vi "HFRR ADV v06.vi"() -> ()   [LabVIEW 2025] (continued)
            n239 = Concatenate Strings("[CH3]" ("string"), w309, " - 20x Gain" ("string"), "\r") -> (w303:string)
            n240 = Concatenate Strings("[CH4]" ("string"), w297, " - 100x Gain" ("string"), "\r") -> (w296:string)
            n241 = String To Path(string="C:\\LAB-IQ\\Image Calibrate v01.dcf") -> (path=w326:path)
            n242 = Concatenate Strings(w313, w312, w303, w296) -> (w311:string)
            n243 = call <vilib>:"Write Characters To File.vi"("append to file? (new file:F)"=FALSE, "character string"=w311, "file path (dialog if empty)"=w326) -> ()  [unwired: 2 in, 1 out]
          }
          frame #2 {
            n244 = String To Path(string="C:\\LAB-IQ\\Image Calibrate v01.dcf") -> (path=w329:path)
            n245 = Open/Create/Replace File ("Open File")(file path (use dialog)=w329) -> (refnum out=w330:refnum<file>)  [unwired: 5 in, 2 out]
            n246 = for {
              N: 4 -> [_]
              tunnel: w330 -> [w336]
              i -> [w332]
              n247 = Read from Text File ("Read File")(file (use dialog)=w336) -> (text=w337:string)  [unwired: 3 in, 3 out]
              n248 = String Subset(string=w337, offset (0)=6, length (rest)=10 ("length (rest)")) -> (substring=w333:string)
              n249 = Fract/Exp String To Number(string=w333) -> (number=w331:dbl)  [unwired: 3 in, 1 out]
              n250 = case shown="3" w332 {
                tunnel: w331 -> [w338 w339 _ w340 _]
                frame 0 {
                  n251 = local write "5x Gain"(w338) -> ()
                }
                frame 1 {
                  n252 = local write "10x Gain"(w339) -> ()
                }
                frame 2 {
                }
                frame 3 {
                  n253 = local write "100x gain"(w340) -> ()
                }
                frame 4, Default {
                }
              }
            }
          }
          frame #3 {
            n254 = call "IMAGE ANALYSIS.vi"("Enum"=POST_ANALYSIS_ENUM."SHOW UI") -> ()  [unwired: 9 in, 2 out]
          }
          frame #4 {
            n255 = Not(x=w343) -> (.not. x?=w342:bool)
            n256 = local write "Save Change"(w342) -> ()
          }
        }
      }
    }
    n257 = local read "Cap Live Image"() -> (w269:bool)
    n258 = local read "SCAR MEASURMENT"() -> (w272:enum32{"Auto Scar", "Manual Scar"})
    n259 = Wait (ms)(milliseconds to wait=u32 250) -> ()  [unwired: 1 out]
    n260 = Equal?(x=w272, y=enum32{"Auto Scar", "Manual Scar"}."Manual Scar" ("SCAR MEASURMENT")) -> (x = y?=w270:bool)
    n261 = And(x=w270, y=w269) -> (x .and. y?=w268:bool)
    n262 = case shown="True" w268 {
      selector: w268 -> [_ w536]
      frame False {
      }
      frame True {
        n263 = stacked-sequence {
          tunnel: [_ _ _ w551 _] -> _
          tunnel: w536 -> [_ _ _ _ w557]
          frame #0 {
            w537 = 0.0
            n264 = local write "Major Axis"(w537) -> ()
            n265 = local write "Minor Axis"(w537) -> ()
            n266 = local write "Average"(w537) -> ()
          }
          frame #1 {
            n267 = call "CAMERA LIVE FEED FGV.vi"("Enum - Menu"=CAMERA_LIVE_FEED_ENUM."CAMERA MINIMIZE") -> ()  [unwired: 9 in, 2 out]
          }
          frame #2 {
            n268 = local read "FILE 3"() -> (w545:string)
            n269 = call <vilib>:"Trim Whitespace.vi"("string"="C:\\LAB-IQ\\images\\") -> ("trimmed string"=w547:string)  [unwired: 1 in]
            n270 = String To Path(string=w547) -> (path=w546:path)
            n271 = Concatenate Strings(w545, ".png" ("string")) -> (w544:string)
            n272 = Build Path(base path=w546, name or relative path=w544) -> (appended path=w542:path)
            n273 = Path To String(path=w542) -> (string=w541:string)
            n274 = call "CAMERA LIVE FEED FGV.vi"("Enum - Menu"=CAMERA_LIVE_FEED_ENUM."CAMERA SAVE", "Image Path"=w541) -> ("error out"=w539:errorcluster)  [unwired: 8 in, 1 out]
            n275 = case shown="No Error" w539 {
              frame No Error {
                n276 = One Button Dialog(message="Image saved successfully") -> ()  [unwired: 1 in, 1 out]
              }
              frame Error {
              }
            }
          }
          frame #3 {
            n277 = call "LIST FILE NAMES.vi"() -> ("error out"=w553:errorcluster, "filenames"=w550:string[])  [unwired: 10 in]
            n278 = call "IMAGE ANALYSIS.vi"("Enum"=POST_ANALYSIS_ENUM."SHOW UI", "error in"=w553) -> ("error out"=w551:errorcluster)  [unwired: 8 in, 1 out]
            n279 = property on="Test File List :" class="CmbBox"("Strings[]"=w550) -> ()  [unwired: 2 in, 2 out]
          }
          frame #4 {
            n280 = Not(x=w557) -> (.not. x?=w556:bool)
            n281 = local write "Zoom Factore"(0.0 ("Zoom Factore")) -> ()
            n282 = local write "Cap Live Image"(w556) -> ()
            n283 = local write "Main Tab"(T2."Adv Scar Report" ("Main Tab")) -> ()
            n284 = local write "Main Dashboard Buttons"(T1."Report" ("Main Dashboard Buttons")) -> ()
            n285 = property on="Cap Live Image" class="Bool (strict)"("BoolText.Text"="Capture Image" ("Boolean Text.Text")) -> ()  [unwired: 2 in, 2 out]
          }
        }
      }
    }
    n286 = local read "change Gain"() -> (w252:bool)
    n287 = local read "Back Square"() -> (w251:bool)
    n288 = case shown="True" w252 {
      selector: w252 -> [_ w280]
      frame False {
      }
      frame True {
        n289 = stacked-sequence {
          tunnel: w280 -> [_ w288]
          frame #0 {
            n290 = local read "Actual (µm)"() -> (w284:dbl)
            n291 = local read "Pixel Value"() -> (w283:dbl)
            n292 = local read "Magnification :"() -> (w282:string)
            n293 = Divide(x=w284, y=w283) -> (x/y=w281:dbl)
            n294 = case shown="\"10x\"" w282 {
              tunnel: w281 -> [w285 w286]
              frame "10x" {
                n295 = local write "10x Gain"(w285) -> ()
              }
              frame "5x", Default {
                n296 = local write "5x Gain"(w286) -> ()
              }
            }
          }
          frame #1 {
            n297 = Not(x=w288) -> (.not. x?=w287:bool)
            n298 = local write "change Gain"(w287) -> ()
          }
        }
      }
    }
    n299 = case shown="True" w251 {
      selector: w251 -> [_ w278]
      frame False {
      }
      frame True {
        n300 = Not(x=w278) -> (.not. x?=w277:bool)
        n301 = local write "Back Square"(w277) -> ()
        n302 = local write "Calibration Tab"(enum32{"Measrument", "Calibrate"}."Measrument" ("Calibration Tab")) -> ()
      }
    }
    n303 = local read "Rectangle Tool"() -> (w263:bool)
    n304 = local read "Clear ROI Tool"() -> (w262:bool)
    n305 = local read "Open Image"() -> (w267:bool)
    n306 = local read "line tool"() -> (w264:bool)
    n307 = local read "OUT"() -> (w265:bool)
    n308 = local read "In"() -> (w266:bool)
    n309 = case shown="True" w267 {
      selector: w267 -> [_ w524]
      tunnel: [w520 w526] -> _
      tunnel: w257 -> [w520 w525]
      frame False {
      }
      frame True {
        n310 = Not(x=w524) -> (.not. x?=w523:bool)
        n311 = local write "Open Image"(w523) -> ()
        n312 = call "IMAGE ANALYSIS.vi"("Enum"=POST_ANALYSIS_ENUM."HIDE UI", "error in"=w525) -> ("error out"=w533:errorcluster)  [unwired: 8 in, 1 out]
        n313 = call "File Dialog"("start path"=path "C:/LAB-IQ/images", "error in"=w533) -> ("selected path"=w522:path, "error out"=w531:errorcluster)  [unwired: 10 in, 2 out]
        "Image path" <- w522
        n314 = call <vilib>:"Clear Errors.vi"("error in (no error)"=w531) -> ("error out"=w530:errorcluster)  [unwired: 5 in, 1 out]
        n315 = call "IMAGE ANALYSIS.vi"("Enum"=POST_ANALYSIS_ENUM."OPEN FILE", "error in"=w530, "File Path"=w522) -> ("error out"=w529:errorcluster)  [unwired: 7 in, 1 out]
        n316 = call <vilib>:"Clear Errors.vi"("error in (no error)"=w529) -> ("error out"=w528:errorcluster)  [unwired: 5 in, 1 out]
        n317 = call "IMAGE ANALYSIS.vi"("Enum"=POST_ANALYSIS_ENUM."SHOW UI", "error in"=w528) -> ("error out"=w526:errorcluster)  [unwired: 8 in, 1 out]
        n318 = local write "Zoom Factore"(100.0 ("Zoom Factore")) -> ()
      }
    }
    n319 = case shown="True" w265 {
      selector: w265 -> [_ w505]
      tunnel: w257 -> [w502 w510]
      tunnel: [w502 w504] -> _
      frame False {
      }
      frame True {
        n320 = Not(x=w505) -> (.not. x?=w503:bool)
        n321 = local read "Zoom Factore"() -> (w508:dbl)
        n322 = local write "OUT"(w503) -> ()
        n323 = call "IMAGE ANALYSIS.vi"("Enum"=POST_ANALYSIS_ENUM."ZOOM OUT", "error in"=w510) -> ("error out"=w504:errorcluster)  [unwired: 8 in, 1 out]
        n324 = Divide(x=w508, y=1.2) -> (x/y=w506:dbl)
        n325 = local write "Zoom Factore"(w506) -> ()
      }
    }
    n326 = case shown="True" w266 {
      selector: w266 -> [_ w514]
      tunnel: w257 -> [w511 w519]
      tunnel: [w511 w512] -> _
      frame False {
      }
      frame True {
        n327 = Not(x=w514) -> (.not. x?=w513:bool)
        n328 = local read "Zoom Factore"() -> (w517:dbl)
        n329 = local write "In"(w513) -> ()
        n330 = call "IMAGE ANALYSIS.vi"("Enum"=POST_ANALYSIS_ENUM."ZOOM IN", "error in"=w519) -> ("error out"=w512:errorcluster)  [unwired: 8 in, 1 out]
        n331 = Multiply(x=w517, y=1.2) -> (x*y=w515:dbl)
        n332 = local write "Zoom Factore"(w515) -> ()
      }
    }
    n333 = case shown="True" w262 {
      selector: w262 -> [_ w486]
      tunnel: w257 -> [w484 w488]
      tunnel: [w484 w487] -> _
      frame False {
      }
      frame True {
        n334 = Not(x=w486) -> (.not. x?=w485:bool)
        n335 = local write "Clear ROI Tool"(w485) -> ()
        n336 = call "IMAGE ANALYSIS.vi"("Enum"=POST_ANALYSIS_ENUM."CLEAR ROI", "error in"=w488) -> ("error out"=w487:errorcluster)  [unwired: 8 in, 1 out]
      }
    }
    n337 = case shown="True" w264 {
      selector: w264 -> [_ w498]
      tunnel: w257 -> [w496 w501]
      tunnel: [w496 w499] -> _
      frame False {
      }
      frame True {
        n338 = Not(x=w498) -> (.not. x?=w497:bool)
        n339 = local write "line tool"(w497) -> ()
        n340 = call "IMAGE ANALYSIS.vi"("Enum"=POST_ANALYSIS_ENUM."DRAW LINE", "error in"=w501) -> ("error out"=w499:errorcluster)  [unwired: 8 in, 1 out]
      }
    }
    n341 = case shown="True" w263 {
      selector: w263 -> [_ w492]
      tunnel: w257 -> [w490 w494]
      tunnel: [w490 w493] -> _
      frame False {
      }
      frame True {
        n342 = Not(x=w492) -> (.not. x?=w491:bool)
        n343 = local write "Rectangle Tool"(w491) -> ()
        n344 = call "IMAGE ANALYSIS.vi"("Enum"=POST_ANALYSIS_ENUM."DRAW REC", "error in"=w494) -> ("error out"=w493:errorcluster)  [unwired: 8 in, 1 out]
      }
    }
    n345 = local read "SCAR MEASURMENT"() -> (w250:enum32{"Auto Scar", "Manual Scar"})
    n346 = local read "Fit to Screen Tool"() -> (w259:bool)
    n347 = local read "Resize Tool"() -> (w258:bool)
    n348 = case shown="\"Manual Scar\"" w250 {
      frame "Auto Scar", Default {
        n349 = property on="Cap Live Image" class="Bool (strict)"("BoolText.Text"="Report" ("Boolean Text.Text")) -> ()  [unwired: 2 in, 2 out]
      }
      frame "Manual Scar" {
        n350 = property on="Cap Live Image" class="Bool (strict)"("BoolText.Text"="Save Image" ("Boolean Text.Text")) -> ()  [unwired: 2 in, 2 out]
      }
    }
    n351 = local read "ROI Color Tool"() -> (w260:bool)
    n352 = local read "Pan Tool"() -> (w261:bool)
    n353 = case shown="True" w261 {
      selector: w261 -> [_ w480]
      tunnel: w257 -> [w478 w482]
      tunnel: [w478 w481] -> _
      frame False {
      }
      frame True {
        n354 = Not(x=w480) -> (.not. x?=w479:bool)
        n355 = call "IMAGE ANALYSIS.vi"("Enum"=POST_ANALYSIS_ENUM."PAN", "error in"=w482) -> ("error out"=w481:errorcluster)  [unwired: 8 in, 1 out]
        n356 = local write "Pan Tool"(w479) -> ()
      }
    }
    n357 = case shown="True" w258 {
      selector: w258 -> [_ w464]
      tunnel: w257 -> [w459 w461]
      tunnel: [w459 w460] -> _
      frame False {
      }
      frame True {
        n358 = Not(x=w464) -> (.not. x?=w463:bool)
        n359 = local write "Resize Tool"(w463) -> ()
        n360 = call "IMAGE ANALYSIS.vi"("Enum"=POST_ANALYSIS_ENUM."RESIZE MODE", "error in"=w461) -> ("error out"=w460:errorcluster)  [unwired: 8 in, 1 out]
      }
    }
    n361 = case shown="True" w259 {
      selector: w259 -> [_ w469]
      tunnel: [w465 w470] -> _
      tunnel: w257 -> [w465 w468]
      frame False {
      }
      frame True {
        n362 = Not(x=w469) -> (.not. x?=w467:bool)
        n363 = local write "Zoom Factore"(100.0 ("Zoom Factore")) -> ()
        n364 = local write "Fit to Screen Tool"(w467) -> ()
        n365 = call "IMAGE ANALYSIS.vi"("Enum"=POST_ANALYSIS_ENUM."FIT", "error in"=w468) -> ("error out"=w470:errorcluster)  [unwired: 8 in, 1 out]
      }
    }
    n366 = case shown="True" w260 {
      selector: w260 -> [_ w475]
      tunnel: [w472 w476] -> _
      tunnel: w257 -> [w472 w473]
      frame False {
      }
      frame True {
        n367 = Not(x=w475) -> (.not. x?=w474:bool)
        n368 = local write "ROI Color Tool"(w474) -> ()
        n369 = call "IMAGE ANALYSIS.vi"("Enum"=POST_ANALYSIS_ENUM."SET ROI COLOR", "error in"=w473) -> ("error out"=w476:errorcluster)  [unwired: 8 in, 1 out]
      }
    }
    n370 = local read "Quit"() -> (w274:bool)
  }
  n371 = property on="Auto Scar Check  2" class="Clust (strict)"("Visible"=FALSE) -> (error out=w1:errorcluster)  [unwired: 2 in, 1 out]
  n372 = while {
    stop <- w560 stop-if-true
    n373 = local read "Image Path"() -> (w563:path)
    n374 = local read "Print 3"() -> (w566:bool)
    n375 = Equal?(x=w563, y=path "") -> (x = y?=w562:bool)
    n376 = Not(x=w562) -> (.not. x?=w561:bool)
    n377 = property on="Print 3" class="Bool (strict)"("Visible"=w561) -> ()  [unwired: 2 in, 2 out]
    n378 = case shown="True" w566 {
      frame False {
        n379 = local write "Rd"(TRUE ("Boolean 7")) -> ()
      }
      frame True {
        n380 = flat-sequence {
          tunnel: [w606] -> w574
          tunnel: [w593] -> w572
          tunnel: [w603] -> w568
          tunnel: w574 -> [w615]
          tunnel: [w615] -> w573
          tunnel: w572 -> [w614]
          tunnel: [w614] -> w571
          tunnel: [w612] -> w570
          tunnel: [w611] -> w569
          tunnel: w568 -> [w611]
          tunnel: w573 -> [w617]
          tunnel: w571 -> [w618]
          tunnel: w570 -> [_]
          tunnel: w569 -> [w616]
          frame #0 {
            n381 = case shown="True" "Rd" {
              frame False {
              }
              frame True {
                n382 = while {
                  tunnel: "abcdefABCDEF" ("string 2") -> [w585]
                  shift-right: [w583] -> w577
                  shift-left: "" -> [w582]
                  i -> [w592]
                  stop <- w591 stop-if-true
                  n383 = Random Number (0-1)() -> (number: 0 to 1=w586:dbl)
                  n384 = Multiply(x=w586, y=62.0) -> (x*y=w588:dbl)
                  n385 = Decrement(x="Length 2") -> (x-1=w581:i16)
                  n386 = To Word Integer(number=w588) -> (16bit integer=w589:i16)
                  n387 = String Subset(string=w585, offset (0)=w589, length (rest)=1 ("length (rest)")) -> (substring=w584:string)
                  n388 = Greater Or Equal?(x=w592, y=w581) -> (x >= y?=w591:bool)
                  n389 = Concatenate Strings(w584, w582) -> (w583:string)
                }
                "String 10" <- w577
                n390 = local write "Rd"(FALSE ("Boolean 7")) -> ()
              }
            }
          }
          frame #1 {
            w604 = "_resized.jpg" ("command line")
            (unwired) ".jpg -resize 320x240 " ("string")
            (unwired) "Choose an Image File" ("prompt")
            # "-resize 1798x425"
            n391 = local read "Image Path"() -> (w598:path)
            n392 = Strip Path(path=w598) -> (stripped path=w593:path, name=w594:string)
            n393 = Match Pattern(string=w594, regular expression=".jpg") -> (before substring=→"before substring 2":string, after substring=→"after substring":string)  [unwired: 1 in, 2 out]
            n394 = Match Pattern(string=w594, regular expression="\\") -> (before substring=w600:string)  [unwired: 1 in, 3 out]
            n395 = Match Pattern(string=w600, regular expression=".jpg") -> (before substring=w599:string)  [unwired: 1 in, 3 out]
            n396 = Concatenate Strings("cmd /c convert " ("string"), w599, ".jpg -resize 320x240  " ("command line"), w599, w604) -> (w607:string)
            n397 = call <vilib>:"System Exec.vi"("run minimized? (F)"=TRUE, "wait until completion? (T)"=TRUE, "working directory"=w593, "command line"=w607) -> ("error out"=w606:errorcluster)  [unwired: 4 in, 3 out]
            "error out 2" <- w606
            n398 = Concatenate Strings(w599, w604) -> (w603:string)
          }
          frame #2 {
            n399 = Wait (ms)(milliseconds to wait=u32 2000 ("millisecond timer value")) -> (millisecond timer value=w612:u32)
          }
          frame #3 {
            n400 = case shown="No Error" w617 {
              tunnel: w618 -> [w621 _]
              tunnel: w616 -> [w619 _]
              frame No Error {
                (unwired) ".jpg" ("string")
                n401 = Path To String(path=w621) -> (string=w625:string)
                n402 = Concatenate Strings(w625, "\\" ("string"), w619) -> (w624:string)
                n403 = String To Path(string=w624) -> (path=w623:path)
                n404 = call <vilib>:"Read JPEG File.vi"("path to JPEG file"=w623) -> ("image data"=w627:T11)  [unwired: 8 in, 2 out]
                "image data" <- w627
                n405 = local write "Print 3"(FALSE ("Print 2")) -> ()
                n406 = call <vilib>:"Draw Flattened Pixmap.vi"("image data"=w627) -> ("new picture"=→"new picture":picture)  [unwired: 8 in]
              }
              frame Error {
              }
            }
          }
        }
      }
    }
    n407 = Wait (ms)(milliseconds to wait=u32 20 ("millisecond timer value")) -> ()  [unwired: 1 out]
    n408 = local read "Quit"() -> (w560:bool)
  }
  n409 = while {
    tunnel: w21 -> [_]
    tunnel: w1 -> [_]
    stop <- w657 stop-if-true
    # "New Adv Logics"
    n410 = local read "Main Tab"() -> (w655:T2)
    n411 = local read "Sign In"() -> (w654:bool)
    n412 = local read "Main Tab"() -> (w636:T2)
    n413 = case shown="\"Adv Scar Report\"" w636 {
      frame "HOME", Default {
        n414 = local read "LIVE FEED MIN TEMP"() -> (w726:bool)
        n415 = local write "LIVE FEED MAX TEMP"(TRUE ("LIVE FEED MAX TEMP")) -> ()
        n416 = local read "CAMERA ROI MIN TEMP"() -> (w724:bool)
        n417 = case shown="True" w726 {
          selector: w726 -> [_ w733]
          frame False {
          }
          frame True {
            n418 = Not(x=w733) -> (.not. x?=w732:bool)
            n419 = local write "LIVE FEED MIN TEMP"(w732) -> ()
            n420 = call "CAMERA LIVE FEED FGV.vi"("Enum - Menu"=CAMERA_LIVE_FEED_ENUM."CAMERA MINIMIZE") -> ()  [unwired: 9 in, 2 out]
          }
        }
        n421 = case shown="True" w724 {
          selector: w724 -> [_ w730]
          frame False {
          }
          frame True {
            n422 = Not(x=w730) -> (.not. x?=w729:bool)
            n423 = local write "CAMERA ROI MIN TEMP"(w729) -> ()
            n424 = call "IMAGE ANALYSIS.vi"("Enum"=POST_ANALYSIS_ENUM."MINIMIZE UI") -> ()  [unwired: 9 in, 2 out]
          }
        }
        n425 = local write "CAMERA ROI MAX TEMP"(TRUE ("CAMERA ROI MAX TEMP")) -> ()
      }
      frame "Test Setup" {
        n426 = local read "LIVE FEED MIN TEMP"() -> (w736:bool)
        n427 = local read "CAMERA ROI MIN TEMP"() -> (w734:bool)
        n428 = local write "LIVE FEED MAX TEMP"(TRUE ("LIVE FEED MAX TEMP")) -> ()
        n429 = case shown="True" w736 {
          selector: w736 -> [_ w743]
          frame False {
          }
          frame True {
            n430 = Not(x=w743) -> (.not. x?=w742:bool)
            n431 = local write "LIVE FEED MIN TEMP"(w742) -> ()
            n432 = call "CAMERA LIVE FEED FGV.vi"("Enum - Menu"=CAMERA_LIVE_FEED_ENUM."CAMERA MINIMIZE") -> ()  [unwired: 9 in, 2 out]
          }
        }
        n433 = case shown="True" w734 {
          selector: w734 -> [_ w740]
          frame False {
          }
          frame True {
            n434 = Not(x=w740) -> (.not. x?=w739:bool)
            n435 = local write "CAMERA ROI MIN TEMP"(w739) -> ()
            n436 = call "IMAGE ANALYSIS.vi"("Enum"=POST_ANALYSIS_ENUM."MINIMIZE UI") -> ()  [unwired: 9 in, 2 out]
          }
        }
        n437 = local write "CAMERA ROI MAX TEMP"(TRUE ("CAMERA ROI MAX TEMP")) -> ()
      }
      frame "Acquire" {
        n438 = local read "LIVE FEED MIN TEMP"() -> (w746:bool)
        n439 = local write "LIVE FEED MAX TEMP"(TRUE ("LIVE FEED MAX TEMP")) -> ()
        n440 = local read "CAMERA ROI MIN TEMP"() -> (w744:bool)
        n441 = case shown="True" w746 {
          selector: w746 -> [_ w753]
          frame False {
          }
          frame True {
            n442 = Not(x=w753) -> (.not. x?=w752:bool)
            n443 = local write "LIVE FEED MIN TEMP"(w752) -> ()
            n444 = call "CAMERA LIVE FEED FGV.vi"("Enum - Menu"=CAMERA_LIVE_FEED_ENUM."CAMERA MINIMIZE") -> ()  [unwired: 9 in, 2 out]
          }
        }
        n445 = case shown="True" w744 {
          selector: w744 -> [_ w750]
          frame False {
          }
          frame True {
            n446 = Not(x=w750) -> (.not. x?=w749:bool)
            n447 = local write "CAMERA ROI MIN TEMP"(w749) -> ()
            n448 = call "IMAGE ANALYSIS.vi"("Enum"=POST_ANALYSIS_ENUM."MINIMIZE UI") -> ()  [unwired: 9 in, 2 out]
          }
        }
        n449 = local write "CAMERA ROI MAX TEMP"(TRUE ("CAMERA ROI MAX TEMP")) -> ()
      }
      frame "Adv Scar" {
        n450 = local read "CAMERA ROI MIN TEMP"() -> (w754:bool)
        n451 = case shown="True" "LIVE FEED MAX TEMP" {
          selector: "LIVE FEED MAX TEMP" -> [_ w766]
          frame False {
          }
          frame True {
            n452 = Not(x=w766) -> (.not. x?=w765:bool)
            n453 = local write "LIVE FEED MAX TEMP"(w765) -> ()
            n454 = call "CAMERA LIVE FEED FGV.vi"("Enum - Menu"=CAMERA_LIVE_FEED_ENUM."CAMERA RESTORE") -> ("error out"=w761:errorcluster)  [unwired: 9 in, 1 out]
            n455 = call "LIST FILE NAMES.vi"("error in (no error)"=w761) -> ("error out"=w762:errorcluster, "filenames"=w763:string[])  [unwired: 9 in]
            n456 = property on="FILE 3" class="CmbBox"(error in=w762, "Strings[]"=w763) -> ()  [unwired: 1 in, 2 out]
          }
        }
        n457 = case shown="True" w754 {
          selector: w754 -> [_ w760]
          frame False {
          }
          frame True {
            n458 = Not(x=w760) -> (.not. x?=w759:bool)
            n459 = local write "CAMERA ROI MIN TEMP"(w759) -> ()
            n460 = call "IMAGE ANALYSIS.vi"("Enum"=POST_ANALYSIS_ENUM."MINIMIZE UI") -> ()  [unwired: 9 in, 2 out]
          }
        }
        n461 = local write "CAMERA ROI MAX TEMP"(TRUE ("CAMERA ROI MAX TEMP")) -> ()
        "LIVE FEED MIN TEMP" <- TRUE ("LIVE FEED MIN TEMP")
      }
      frame "Adv Scar Report" {
        n462 = local read "CAMERA ROI MAX TEMP"() -> (w767:bool)
        n463 = local read "LIVE FEED MIN TEMP"() -> (w769:bool)
        n464 = local write "LIVE FEED MAX TEMP"(TRUE ("LIVE FEED MAX TEMP")) -> ()
        n465 = case shown="True" w769 {
          selector: w769 -> [_ w778]
          frame False {
          }
          frame True {
            n466 = Not(x=w778) -> (.not. x?=w777:bool)
            n467 = local write "LIVE FEED MIN TEMP"(w777) -> ()
            n468 = call "CAMERA LIVE FEED FGV.vi"("Enum - Menu"=CAMERA_LIVE_FEED_ENUM."CAMERA MINIMIZE") -> ()  [unwired: 9 in, 2 out]
          }
        }
        n469 = case shown="True" w767 {
          selector: w767 -> [_ w775]
          frame False {
          }
          frame True {
            n470 = Not(x=w775) -> (.not. x?=w773:bool)
            n471 = local write "CAMERA ROI MAX TEMP"(w773) -> ()
            n472 = call "IMAGE ANALYSIS.vi"("Enum"=POST_ANALYSIS_ENUM."SHOW UI") -> ("error out"=w772:errorcluster)  [unwired: 9 in, 1 out]
            n473 = call "LIST FILE NAMES.vi"("error in (no error)"=w772) -> ("filenames"=w771:string[])  [unwired: 9 in, 1 out]
            n474 = property on="Test File List :" class="CmbBox"("Strings[]"=w771) -> ()  [unwired: 2 in, 2 out]
          }
        }
        n475 = local write "CAMERA ROI MIN TEMP"(TRUE ("CAMERA ROI MIN TEMP")) -> ()
      }
      frame "Compare Files" {
        n476 = local read "LIVE FEED MIN TEMP"() -> (w781:bool)
        n477 = local write "LIVE FEED MAX TEMP"(TRUE ("LIVE FEED MAX TEMP")) -> ()
        n478 = local read "CAMERA ROI MIN TEMP"() -> (w779:bool)
        n479 = case shown="True" w781 {
          selector: w781 -> [_ w788]
          frame False {
          }
          frame True {
            n480 = Not(x=w788) -> (.not. x?=w787:bool)
            n481 = local write "LIVE FEED MIN TEMP"(w787) -> ()
            n482 = call "CAMERA LIVE FEED FGV.vi"("Enum - Menu"=CAMERA_LIVE_FEED_ENUM."CAMERA MINIMIZE") -> ()  [unwired: 9 in, 2 out]
          }
        }
        n483 = case shown="True" w779 {
          selector: w779 -> [_ w785]
          frame False {
          }
          frame True {
            n484 = Not(x=w785) -> (.not. x?=w784:bool)
            n485 = local write "CAMERA ROI MIN TEMP"(w784) -> ()
            n486 = call "IMAGE ANALYSIS.vi"("Enum"=POST_ANALYSIS_ENUM."MINIMIZE UI") -> ()  [unwired: 9 in, 2 out]
          }
        }
        n487 = local write "CAMERA ROI MAX TEMP"(TRUE ("CAMERA ROI MAX TEMP")) -> ()
      }
      frame "About" {
        n488 = local read "LIVE FEED MIN TEMP"() -> (w791:bool)
        n489 = local write "LIVE FEED MAX TEMP"(TRUE ("LIVE FEED MAX TEMP")) -> ()
        n490 = local read "CAMERA ROI MIN TEMP"() -> (w789:bool)
        n491 = case shown="True" w791 {
          selector: w791 -> [_ w798]
          frame False {
          }
          frame True {
            n492 = Not(x=w798) -> (.not. x?=w797:bool)
            n493 = local write "LIVE FEED MIN TEMP"(w797) -> ()
            n494 = call "CAMERA LIVE FEED FGV.vi"("Enum - Menu"=CAMERA_LIVE_FEED_ENUM."CAMERA MINIMIZE") -> ()  [unwired: 9 in, 2 out]
          }
        }
        n495 = case shown="True" w789 {
          selector: w789 -> [_ w795]
          frame False {
          }
          frame True {
            n496 = Not(x=w795) -> (.not. x?=w794:bool)
            n497 = local write "CAMERA ROI MIN TEMP"(w794) -> ()
            n498 = call "IMAGE ANALYSIS.vi"("Enum"=POST_ANALYSIS_ENUM."MINIMIZE UI") -> ()  [unwired: 9 in, 2 out]
          }
        }
        n499 = local write "CAMERA ROI MIN TEMP"(TRUE ("CAMERA ROI MIN TEMP")) -> ()
      }
      frame "Advance" {
        n500 = local read "LIVE FEED MIN TEMP"() -> (w801:bool)
        n501 = local write "LIVE FEED MAX TEMP"(TRUE ("LIVE FEED MAX TEMP")) -> ()
        n502 = local read "CAMERA ROI MIN TEMP"() -> (w799:bool)
        n503 = case shown="True" w801 {
          selector: w801 -> [_ w808]
          frame False {
          }
          frame True {
            n504 = Not(x=w808) -> (.not. x?=w807:bool)
            n505 = local write "LIVE FEED MIN TEMP"(w807) -> ()
            n506 = call "CAMERA LIVE FEED FGV.vi"("Enum - Menu"=CAMERA_LIVE_FEED_ENUM."CAMERA MINIMIZE") -> ()  [unwired: 9 in, 2 out]
          }
        }
        n507 = local write "CAMERA ROI MAX TEMP"(TRUE ("CAMERA ROI MAX TEMP")) -> ()
        n508 = case shown="True" w799 {
          selector: w799 -> [_ w805]
          frame False {
          }
          frame True {
            n509 = Not(x=w805) -> (.not. x?=w804:bool)
            n510 = local write "CAMERA ROI MIN TEMP"(w804) -> ()
            n511 = call "IMAGE ANALYSIS.vi"("Enum"=POST_ANALYSIS_ENUM."MINIMIZE UI") -> ()  [unwired: 9 in, 2 out]
          }
        }
      }
      frame "Mooha" {
        n512 = local read "LIVE FEED MIN TEMP"() -> (w811:bool)
        n513 = local write "LIVE FEED MAX TEMP"(TRUE ("LIVE FEED MAX TEMP")) -> ()
        n514 = local read "CAMERA ROI MIN TEMP"() -> (w809:bool)
        n515 = case shown="True" w811 {
          selector: w811 -> [_ w818]
          frame False {
          }
          frame True {
            n516 = Not(x=w818) -> (.not. x?=w817:bool)
            n517 = local write "LIVE FEED MIN TEMP"(w817) -> ()
            n518 = call "CAMERA LIVE FEED FGV.vi"("Enum - Menu"=CAMERA_LIVE_FEED_ENUM."CAMERA MINIMIZE") -> ()  [unwired: 9 in, 2 out]
          }
        }
        n519 = local write "CAMERA ROI MAX TEMP"(TRUE ("CAMERA ROI MAX TEMP")) -> ()
        n520 = case shown="True" w809 {
          selector: w809 -> [_ w815]
          frame False {
          }
          frame True {
            n521 = Not(x=w815) -> (.not. x?=w814:bool)
            n522 = local write "CAMERA ROI MIN TEMP"(w814) -> ()
            n523 = call "IMAGE ANALYSIS.vi"("Enum"=POST_ANALYSIS_ENUM."MINIMIZE UI") -> ()  [unwired: 9 in, 2 out]
          }
        }
      }
    }
    n524 = case shown="True" "sign in temp" {
      frame False {
      }
      frame True {
        w661 = 1 ("y")
        n525 = local read "USERNAME"() -> (w667:string)
        n526 = local read "USER ID"() -> (w664:string)
        n527 = call <vilib>:"Trim Whitespace.vi"("string"=w667) -> ("trimmed string"=w666:string)  [unwired: 1 in]
        n528 = call <vilib>:"Trim Whitespace.vi"("string"=w664) -> ("trimmed string"=w665:string)  [unwired: 1 in]
        n529 = String Length(string=w666) -> (length=w663:i32)
        n530 = String Length(string=w665) -> (length=w662:i32)
        n531 = Greater?(x=w663, y=w661) -> (0:w660:bool)
        n532 = Greater?(x=w662, y=w661) -> (0:w659:bool)
        n533 = And(x=w660, y=w659) -> (x .and. y?=w658:bool)
        n534 = case shown="True" w658 {
          frame False {
            n535 = property on="Sign In" class="Bool (strict)"("DisabledEnum"=T14."Disabled" ("Disabled")) -> ()  [unwired: 2 in, 2 out]
          }
          frame True {
            n536 = property on="Sign In" class="Bool (strict)"("DisabledEnum"=T14."Enabled" ("Disabled")) -> ()  [unwired: 2 in, 2 out]
          }
        }
      }
    }
    n537 = local read "Air Temperature"() -> (w644:bool)
    n538 = local read "Coefficient Of Friction"() -> (w645:bool)
    n539 = local read "Humidity"() -> (w643:bool)
    n540 = case shown="\"HOME\"" w655 {
      frame "HOME" {
        n541 = local write "main tab sub"(enum32{"Page 1", "Page 2"}."Page 1" ("main tab sub")) -> ()
      }
      frame Default {
        n542 = local write "main tab sub"(enum32{"Page 1", "Page 2"}."Page 2" ("main tab sub")) -> ()
      }
    }
    n543 = case shown="True" w654 {
      selector: w654 -> [_ w907]
      frame False {
      }
      frame True {
        n544 = Not(x=w907) -> (.not. x?=w906:bool)
        n545 = local write "Sign In"(w906) -> ()
        n546 = local write "Main Dashboard Buttons"(T1."Test Setup" ("Main Dashboard Buttons")) -> ()
      }
    }
    n547 = case shown="\"Numeric Display\", Default" "Num/Graph" {
      frame "Numeric Display", Default {
        n548 = property on="Single/Multiple" class="RadioBtnsControl (strict)"("Visible"=FALSE) -> ()  [unwired: 2 in, 2 out]
        n549 = property on="Single - Graph" class="Ring (strict)"("Visible"=FALSE) -> ()  [unwired: 2 in, 2 out]
        n550 = local write "Main Tab Display"(T4."Dashboard 1" ("Main Tab Display")) -> ()
      }
      frame "Graph Display" {
        n551 = property on="Single/Multiple" class="RadioBtnsControl (strict)"("Visible"=TRUE) -> ()  [unwired: 2 in, 2 out]
        n552 = case shown="\"Multiple\"" "Single/Multiple" {
          frame "Single ", Default {
            n553 = property on="Single - Graph" class="Ring (strict)"("Visible"=TRUE) -> ()  [unwired: 2 in, 2 out]
            n554 = local write "Main Tab Display"(T4."Dashboard 3" ("Main Tab Display")) -> ()
          }
          frame "Multiple" {
            n555 = property on="Single - Graph" class="Ring (strict)"("Visible"=FALSE) -> ()  [unwired: 2 in, 2 out]
            n556 = local write "Main Tab Display"(T4."Dashboard 2" ("Main Tab Display")) -> ()
          }
        }
      }
    }
    n557 = local read "Stroke"() -> (w642:bool)
    n558 = local read "USERNAME"() -> (w648:string)
    n559 = local read "USER ID"() -> (w647:string)
    n560 = case shown="True" w645 {
      selector: w645 -> [_ w858]
      frame False {
      }
      frame True {
        n561 = Not(x=w858) -> (.not. x?=w857:bool)
        n562 = local write "Coefficient Of Friction"(w857) -> ()
        n563 = local write "Tab Control 2"(T6."Coefficient Of Friction" ("Tab Control 2")) -> ()
      }
    }
    n564 = case shown="True" w644 {
      selector: w644 -> [_ w855]
      frame False {
      }
      frame True {
        n565 = Not(x=w855) -> (.not. x?=w853:bool)
        n566 = local write "Air Temperature"(w853) -> ()
        n567 = local write "Tab Control 2"(T6."Air Temperature" ("Tab Control 2")) -> ()
      }
    }
    n568 = local write "Operator ID"(w647) -> ()
    n569 = case shown="True" w642 {
      selector: w642 -> [_ w849]
      frame False {
      }
      frame True {
        n570 = Not(x=w849) -> (.not. x?=w847:bool)
        n571 = local write "Stroke"(w847) -> ()
        n572 = local write "Tab Control 2"(T6."Stroke" ("Tab Control 2")) -> ()
      }
    }
    n573 = local write "tested by"(w648) -> ()
    n574 = case shown="True" w643 {
      selector: w643 -> [_ w852]
      frame False {
      }
      frame True {
        n575 = Not(x=w852) -> (.not. x?=w850:bool)
        n576 = local write "Humidity"(w850) -> ()
        n577 = local write "Tab Control 2"(T6."Humidity" ("Tab Control 2")) -> ()
      }
    }
    n578 = case shown="\"Imaging\"" "Main Dashboard Buttons" {
      tunnel: [T2."HOME" ("Main Tab") T2."Test Setup" ("Main Tab") T2."Acquire" ("Main Tab") T2."Adv Scar" ("Main Tab") T2."Adv Scar Report" ("Main Tab") T2."Compare Files" ("Main Tab") T2."About" ("Main Tab")] -> w652
      frame "Home", Default {
      }
      frame "Test Setup" {
      }
      frame "Dashboard" {
      }
      frame "Imaging" {
      }
      frame "Report" {
      }
      frame "Analysis" {
      }
      frame "About" {
      }
    }
    n579 = Wait (ms)(milliseconds to wait=u32 100) -> ()  [unwired: 1 out]
    n580 = local read "Main Tab Display"() -> (w646:T4)
    n581 = local write "Main Tab"(w652) -> ()
    n582 = case shown="\"Dashboard 3\"" w646 {
      frame "Dashboard 1", Default {
        n583 = property on="Reset Graph" class="Bool (strict)"("Visible"=FALSE) -> ()  [unwired: 2 in, 2 out]
      }
      frame "Dashboard 2" {
        n584 = property on="Reset Graph" class="Bool (strict)"("Visible"=TRUE) -> ()  [unwired: 2 in, 2 out]
      }
      frame "Dashboard 3" {
        n585 = property on="Reset Graph" class="Bool (strict)"("Visible"=TRUE) -> ()  [unwired: 2 in, 2 out]
      }
    }
    n586 = local read "SCAR MEASURMENT"() -> (w634:enum32{"Auto Scar", "Manual Scar"})
    n587 = local read "Humidity"() -> (w649:bool)
    n588 = local read "Cap Live Image"() -> (w631:bool)
    n589 = local read "Sample Temperature"() -> (w641:bool)
    n590 = local read "Air Temp vs Humidity"() -> (w639:bool)
    n591 = local read "Frequency"() -> (w640:bool)
    n592 = Equal?(x=w634, y=enum32{"Auto Scar", "Manual Scar"}."Auto Scar" ("SCAR MEASURMENT")) -> (x = y?=w630:bool)
    n593 = case shown="True" w649 {
      frame False {
        n594 = local write "Humidity On Command"(TRUE ("Humidity On Command")) -> ()
        n595 = case shown="True" "Humidity Off Command" {
          selector: "Humidity Off Command" -> [_ w871]
          frame False {
          }
          frame True {
            n596 = Not(x=w871) -> (.not. x?=w870:bool)
            n597 = local write "Humidity Off Command"(w870) -> ()
            n598 = local read "WriteHumidity"() -> (w868:string[])
            n599 = local read "EVENT LOG"() -> (w865:string)
            n600 = call "Event Log.vi"("Content"="Humidity Control Off" ("string"), "EVENT LOG"=w865) -> ("EVENT LOG"=w866:string)  [unwired: 8 in, 1 out]
            n601 = Insert Into Array(array=w868, new element="R;1" ("new element/subarray")) -> (w869:string[])  [unwired: 1 in]
            n602 = local write "EVENT LOG"(w866) -> ()
            n603 = local write "WriteHumidity"(w869) -> ()
          }
        }
      }
      frame True {
        n604 = case shown="True" "Humidity On Command" {
          selector: "Humidity On Command" -> [_ w884]
          frame False {
          }
          frame True {
            n605 = local read "Set Rh"() -> (w879:dbl)
            n606 = Not(x=w884) -> (.not. x?=w883:bool)
            n607 = local write "Humidity On Command"(w883) -> ()
            n608 = Number To Fractional String(number=w879, precision (6)=i16 2) -> (F-format string=w876:string)  [unwired: 2 in]
            n609 = local read "WriteHumidity"() -> (w881:string[])
            n610 = Concatenate Strings("M;" ("new element/subarray"), w876) -> (w880:string)
            n611 = Concatenate Strings("Humidity Set to : " ("string"), w876, "% RH" ("string")) -> (w874:string)
            n612 = Insert Into Array(array=w881, new element=w880) -> (w882:string[])  [unwired: 1 in]
            n613 = disable-structure shown="Enabled" {
              disable-tunnel: w874 -> [_ _]
              frame Enabled {
                n614 = local read "EVENT LOG"() -> (w887:string)
                n615 = call "Event Log.vi"("Content"="Humidity Control On", "EVENT LOG"=w887) -> ("EVENT LOG"=w888:string)  [unwired: 8 in, 1 out]
                n616 = local write "EVENT LOG"(w888) -> ()
              }
              frame Disabled {
              }
            }
            n617 = local write "WriteHumidity"(w882) -> ()
          }
        }
        n618 = local write "Humidity Off Command"(TRUE ("Humidity Off Command")) -> ()
      }
    }
    n619 = local read "TEST STANDARD"() -> (w637:T3)
    n620 = And(x=w631, y=w630) -> (x .and. y?=w632:bool)
    n621 = case shown="True" w632 {
      selector: w632 -> [_ w679]
      tunnel: errorcluster {"status"=FALSE, "code"=0, "source"=""} ("error in (no error) 3") -> [_ w680]
      frame False {
      }
      frame True {
        n622 = stacked-sequence {
          tunnel: w680 -> [_ _ _ _ _ _ _ w722]
          tunnel: w679 -> [_ _ _ _ _ w707 _ _]
          frame #0 {
            n623 = call "CAMERA LIVE FEED FGV.vi"("Enum - Menu"=CAMERA_LIVE_FEED_ENUM."CAMERA MINIMIZE") -> ()  [unwired: 9 in, 2 out]
          }
          frame #1 {
            n624 = property on="Auto Scar Check  2" class="Clust (strict)"("Visible"=TRUE) -> ()  [unwired: 2 in, 2 out]
          }
          frame #2 {
            n625 = String To Path(string="C:\\LAB-IQ\\Image Calibrate v01.dcf") -> (path=w685:path)
            n626 = Open/Create/Replace File ("Open File")(file path (use dialog)=w685) -> (refnum out=w686:refnum<file>)  [unwired: 5 in, 2 out]
            n627 = for {
              N: 4 -> [_]
              tunnel: w686 -> [w692]
              i -> [w688]
              n628 = Read from Text File ("Read File")(file (use dialog)=w692) -> (text=w693:string)  [unwired: 3 in, 3 out]
              n629 = String Subset(string=w693, offset (0)=6, length (rest)=10 ("length (rest)")) -> (substring=w689:string)
              n630 = Fract/Exp String To Number(string=w689) -> (number=w687:dbl)  [unwired: 3 in, 1 out]
              n631 = case shown="0" w688 {
                tunnel: w687 -> [w694 w695 _ w696 _]
                frame 0 {
                  "5x Gain" <- w694
                }
                frame 1 {
                  "10x Gain" <- w695
                }
                frame 2 {
                }
                frame 3 {
                  "100x gain" <- w696
                }
                frame 4, Default {
                }
              }
            }
          }
          frame #3 {
            n632 = local read "FILE 3"() -> (w702:string)
            n633 = call <vilib>:"Trim Whitespace.vi"("string"="C:\\LAB-IQ\\images\\") -> ("trimmed string"=w704:string)  [unwired: 1 in]
            n634 = String To Path(string=w704) -> (path=w703:path)
            n635 = Concatenate Strings(w702, ".png" ("string")) -> (w701:string)
            n636 = Build Path(base path=w703, name or relative path=w701) -> (appended path=w699:path)
            "Image path" <- w699
            n637 = Path To String(path=w699) -> (string=w698:string)
            n638 = call "CAMERA LIVE FEED FGV.vi"("Enum - Menu"=CAMERA_LIVE_FEED_ENUM."CAMERA SAVE", "Image Path"=w698) -> ()  [unwired: 8 in, 2 out]
          }
          frame #4 {
            n639 = One Button Dialog(message="Image saved successfully") -> ()  [unwired: 1 in, 1 out]
          }
          frame #5 {
            n640 = local read "Magnification len live scar"() -> (w718:string)
            n641 = Not(x=w707) -> (.not. x?=w708:bool)
            n642 = local write "Cap Live Image"(w708) -> ()
            n643 = case shown="\"5x\", Default" w718 {
              tunnel: [w719 w720] -> w717
              frame "5x", Default {
                n644 = local read "5x Gain"() -> (w719:dbl)
              }
              frame "10x" {
                # "5x"
                n645 = local read "10x Gain"() -> (w720:dbl)
              }
            }
            n646 = local read "Image path"() -> (w716:path)
            n647 = local read "FILE 3"() -> (w709:string)
            n648 = call "EDGE DETCTION.vi"("GAIN VALUE"=w717, "Image Path"=w716) -> ("error out"=w715:errorcluster, "return value"=w714:cluster{string, string, dbl, dbl, dbl})  [unwired: 8 in]
            n649 = Bundle By Name(cluster=T17 {"File Name"="", "Test Method"="", "Operator"="", "Fuel Description"="", "Date and time"=""} ("Main Ref"), "File Name"=w709) -> (w710:T17)
            n650 = call "duf file read.vi"("error in (no error)"=w715, "Main Ref"=w710) -> ("error out"=w713:errorcluster, "Main Ref 2"=w711:T17)  [unwired: 8 in]
            n651 = call "EDGE DETECTION REPORT.vi"("error in (no error)"=w713, "return value 2"=w714, "Main Ref"=w711) -> ()  [unwired: 8 in, 1 out]
          }
          frame #6 {
            n652 = property on="Auto Scar Check  2" class="Clust (strict)"("Visible"=FALSE) -> ()  [unwired: 2 in, 2 out]
          }
          frame #7 {
            n653 = call "CAMERA LIVE FEED FGV.vi"("Enum - Menu"=CAMERA_LIVE_FEED_ENUM."CAMERA RESTORE", "error in (no error)"=w722) -> ()  [unwired: 8 in, 2 out]
          }
        }
      }
    }
    n654 = local read "Heater Button"() -> (w638:bool)
    n655 = case shown="True" w640 {
      selector: w640 -> [_ w843]
      frame False {
      }
      frame True {
        n656 = Not(x=w843) -> (.not. x?=w841:bool)
        n657 = local write "Frequency"(w841) -> ()
        n658 = local write "Tab Control 2"(T6."Frequency" ("Tab Control 2")) -> ()
      }
    }
    n659 = case shown="True" w639 {
      selector: w639 -> [_ w840]
      frame False {
      }
      frame True {
        n660 = Not(x=w840) -> (.not. x?=w838:bool)
        n661 = local write "Air Temp vs Humidity"(w838) -> ()
        n662 = local write "Tab Control 2"(T6."Air Temp vs Rh" ("Tab Control 2")) -> ()
      }
    }
    n663 = case shown="True" w641 {
      selector: w641 -> [_ w846]
      frame False {
      }
      frame True {
        n664 = Not(x=w846) -> (.not. x?=w844:bool)
        n665 = local write "Sample Temperature"(w844) -> ()
        n666 = local write "Tab Control 2"(T6."Sample Temperature" ("Tab Control 2")) -> ()
      }
    }
    n667 = case shown="\"Custom\"" w637 {
      frame "ASTM D6079", Default {
        w819 = "ASTM D6079 TEST CONDITIONS" ("Standard 2")
        n668 = local write "Standard 2"(w819) -> ()
        n669 = local write "Standard"(w819) -> ()
      }
      frame "ISO 12156" {
        w820 = "ISO 12156 TEST CONDITIONS" ("Standard 2")
        n670 = local write "Standard 2"(w820) -> ()
        n671 = local write "Standard"(w820) -> ()
      }
      frame "CEC F-096-A-06" {
        w821 = "CEC F-096-A-06 TEST CONDITIONS" ("Standard 2")
        n672 = local write "Standard 2"(w821) -> ()
        n673 = local write "Standard"(w821) -> ()
      }
      frame "Custom" {
        w822 = "CUSTOM TEST CONDITIONS" ("Standard 2")
        n674 = local write "Standard 2"(w822) -> ()
        n675 = local write "Standard"(w822) -> ()
      }
    }
    n676 = case shown="True" w638 {
      frame False {
        n677 = local write "Temperature On Command"(TRUE ("Temperature On Command")) -> ()
        n678 = case shown="True" "Temperature Off Command" {
          selector: "Temperature Off Command" -> [_ w826]
          frame False {
          }
          frame True {
            n679 = Not(x=w826) -> (.not. x?=w825:bool)
            n680 = local read "EVENT LOG"() -> (w829:string)
            n681 = local write "Temperature Off Command"(w825) -> ()
            n682 = call "Event Log.vi"("Content"="Heater Off", "EVENT LOG"=w829) -> ("EVENT LOG"=w828:string)  [unwired: 8 in, 1 out]
            n683 = local write "EVENT LOG"(w828) -> ()
          }
        }
      }
      frame True {
        n684 = local write "Temperature Off Command"(TRUE ("Temperature Off Command")) -> ()
        n685 = case shown="True" "Temperature On Command" {
          selector: "Temperature On Command" -> [_ w833]
          frame False {
          }
          frame True {
            n686 = Not(x=w833) -> (.not. x?=w832:bool)
            n687 = local write "Temperature On Command"(w832) -> ()
            n688 = disable-structure shown="Enabled" {
              disable-tunnel: "Heater On" -> [w835 _]
              frame Enabled {
                n689 = local read "EVENT LOG"() -> (w836:string)
                n690 = call "Event Log.vi"("Content"=w835, "EVENT LOG"=w836) -> ("EVENT LOG"=w837:string)  [unwired: 8 in, 1 out]
                n691 = local write "EVENT LOG"(w837) -> ()
              }
              frame Disabled {
              }
            }
          }
        }
      }
    }
    n692 = local read "Main Tab"() -> (w629:T2)
    n693 = case shown="\"Acquire\"" w629 {
      frame "HOME", Default {
        w670 = T14."Enabled" ("Disabled")
        n694 = property on="Imaging" class="Bool (strict)"("DisabledEnum"=w670) -> ()  [unwired: 2 in, 2 out]
        n695 = property on="Dashboard" class="Bool (strict)"("DisabledEnum"=w670) -> ()  [unwired: 2 in, 2 out]
        n696 = property on="About" class="Bool (strict)"("DisabledEnum"=w670) -> ()  [unwired: 2 in, 2 out]
        n697 = property on="Test Setup" class="Bool (strict)"("DisabledEnum"=w670) -> ()  [unwired: 2 in, 2 out]
        n698 = property on="Analysis" class="Bool (strict)"("DisabledEnum"=w670) -> ()  [unwired: 2 in, 2 out]
        n699 = property on="Main Dashboard Buttons" class="RadioBtnsControl (strict)"("DisabledEnum"=w670) -> ()  [unwired: 2 in, 2 out]
        n700 = property on="Home" class="Bool (strict)"("DisabledEnum"=w670) -> ()  [unwired: 2 in, 2 out]
        n701 = property on="Report" class="Bool (strict)"("DisabledEnum"=w670) -> ()  [unwired: 2 in, 2 out]
      }
      frame "Test Setup" {
        w671 = T14."Enabled" ("Disabled")
        n702 = property on="Dashboard" class="Bool (strict)"("DisabledEnum"=T14."Disabled" ("Disabled")) -> ()  [unwired: 2 in, 2 out]
        n703 = property on="Imaging" class="Bool (strict)"("DisabledEnum"=w671) -> ()  [unwired: 2 in, 2 out]
        n704 = property on="About" class="Bool (strict)"("DisabledEnum"=w671) -> ()  [unwired: 2 in, 2 out]
        n705 = property on="Test Setup" class="Bool (strict)"("DisabledEnum"=w671) -> ()  [unwired: 2 in, 2 out]
        n706 = property on="Analysis" class="Bool (strict)"("DisabledEnum"=w671) -> ()  [unwired: 2 in, 2 out]
        n707 = property on="Home" class="Bool (strict)"("DisabledEnum"=w671) -> ()  [unwired: 2 in, 2 out]
        n708 = property on="Report" class="Bool (strict)"("DisabledEnum"=w671) -> ()  [unwired: 2 in, 2 out]
      }
      frame "Acquire" {
        n709 = local read "RUN"() -> (w673:bool)
        n710 = case shown="True" w673 {
          tunnel: [T14."Enabled" ("Disabled") T14."Disabled" ("Disabled")] -> w676
          frame False {
          }
          frame True {
          }
        }
        n711 = property on="Test Setup" class="Bool (strict)"("DisabledEnum"=T14."Disabled" ("Disabled")) -> ()  [unwired: 2 in, 2 out]
        n712 = property on="About" class="Bool (strict)"("DisabledEnum"=T14."Enabled" ("Disabled")) -> ()  [unwired: 2 in, 2 out]
        n713 = property on="Imaging" class="Bool (strict)"("DisabledEnum"=w676) -> ()  [unwired: 2 in, 2 out]
        n714 = property on="Dashboard" class="Bool (strict)"("DisabledEnum"=w676) -> ()  [unwired: 2 in, 2 out]
        n715 = property on="Analysis" class="Bool (strict)"("DisabledEnum"=w676) -> ()  [unwired: 2 in, 2 out]
        n716 = property on="Home" class="Bool (strict)"("DisabledEnum"=w676) -> ()  [unwired: 2 in, 2 out]
        n717 = property on="Report" class="Bool (strict)"("DisabledEnum"=w676) -> ()  [unwired: 2 in, 2 out]
      }
    }
    n718 = local read "Quit"() -> (w657:bool)
    "Single" <- "Single - Graph"
  }
  n719 = disable-structure shown="Disabled" {
    disable-tunnel: [w911 _] -> w27
    disable-tunnel: _ -> [w910 _]
    frame Disabled {
      n720 = while {
        tunnel: w910 -> [_]
        tunnel: [w912] -> w911
        tunnel: [w913] -> _
        i -> [w913]
        stop <- w912 stop-if-true
        w929 = u16 10 items=["1.0"=10, "1.5"=15, "2.0"=20] ("stop bits (10: 1 bit)")
        n721 = Wait (ms)(milliseconds to wait=u32 10) -> ()  [unwired: 1 out]
        n722 = call-poly "VISA Configure Serial Port"("VISA resource name"=refnum<visa-resource-name> "ASRL1::INSTR" ("COM PORT"), "timeout (10sec)"=u32 10, "baud rate (9600)"=u32 57600, "data bits (8)"=u16 8, "stop bits (10: 1 bit)"=w929) -> ("VISA resource name out"=w915:refnum<visa-resource-name>, "error out"=w924:errorcluster)  [unwired: 9 in]
        n723 = VISA Read(VISA resource name=w915, byte count=u32 2 ("byte count (0)")) -> (read buffer=w923:string)  [unwired: 1 in, 3 out]
        n724 = String Subset(string=w923, offset (0)=0, length (rest)=2 ("length (rest)")) -> (substring=w922:string)
        n725 = Match Pattern(string=w922, regular expression="<>") -> (offset past match=w919:i32)  [unwired: 1 in, 3 out]
        n726 = Greater Or Equal?(x=w919, y=0) -> (x >= y?=w914:bool)
        n727 = case shown="True" w914 {
          tunnel: w915 -> [_ w933]
          tunnel: w924 -> [_ w932]
          frame False {
          }
          frame True {
            n728 = VISA Read(VISA resource name=w933, byte count=u32 32 ("byte count (0)"), error in (no error)=w932) -> (read buffer=w931:string)  [unwired: 3 out]
            n729 = String Subset(string=w931, offset (0)=0, length (rest)=8 ("length (rest)")) -> (substring=w935:string)
            n730 = String Subset(string=w931, offset (0)=8, length (rest)=8 ("length (rest)")) -> (substring=w936:string)
            n731 = Decimal String To Number(string=w936) -> (number=w943:i32)  [unwired: 2 in, 1 out]
            n732 = Decimal String To Number(string=w935) -> (number=w939:i32)  [unwired: 2 in, 1 out]
            n733 = Divide(x=w943, y=10000) -> ()  [unwired: 1 out]
            n734 = Divide(x=w939, y=1000000) -> ()  [unwired: 1 out]
          }
        }
        n735 = local read "Quit"() -> (w912:bool)
      }
    }
    frame Enabled {
    }
  }
  n736 = local write "Err Count"(0 ("Err Count")) -> ()
  n737 = local write "FRICVALZ"(0.0 ("FRICVALZ")) -> ()
  n738 = Tick Count (ms)() -> (millisecond timer value=w40:u32)
  n739 = while {
    shift-right: [w962] -> w44
    shift-left: _ -> [w951]
    shift-right: [w961] -> w43
    shift-left: errorcluster {"status"=TRUE, "code"=0, "source"="Init"} ("error IO") -> [w953]
    shift-right: [w959] -> _
    shift-left: w40 -> [w960]
    tunnel: [w945] -> w31
    tunnel: [w958] -> _
    i -> [w958]
    stop <- w945 stop-if-true
    n740 = local read "Com Port 1"() -> (w952:refnum<visa-resource-name>)
    n741 = local read "Port 1a"() -> (w954:bool)
    n742 = local read "Port 3"() -> (w955:bool)
    n743 = Not Equal?(x=w952, y=w951) -> (x != y?=w950:bool)
    n744 = Or(x=w955, y=w954) -> (x .or. y?=w957:bool)
    n745 = Unbundle(w953) -> ("status"=→"Port 3":bool)  [unwired: 2 out]
    n746 = flat-sequence {
      tunnel: [w965] -> w949
      tunnel: w953 -> [w965]
      frame #0 {
        n747 = Wait (ms)(milliseconds to wait=u32 200) -> ()  [unwired: 1 out]
      }
    }
    n748 = case shown="False" w957 {
      frame False {
        w967 = FALSE ("Visible")
        n749 = property on="Port 1a" class="Bool (strict)"("Visible"=w967) -> ()  [unwired: 2 in, 2 out]
        n750 = property on="Port 3" class="Bool (strict)"("Visible"=w967) -> ()  [unwired: 2 in, 2 out]
      }
      frame True {
        w968 = TRUE ("Visible")
        n751 = property on="Port 1a" class="Bool (strict)"("Visible"=w968) -> ()  [unwired: 2 in, 2 out]
        n752 = property on="Port 3" class="Bool (strict)"("Visible"=w968) -> ()  [unwired: 2 in, 2 out]
      }
    }
    n753 = local read "Re-Initialise"() -> (w946:bool)
    n754 = Or(x=w950, y=w946) -> (x .or. y?=w947:bool)
    n755 = case shown="True" w947 {
      tunnel: [w963 errorcluster {"status"=TRUE, "code"=0, "source"="Init"} ("error out")] -> w948
      tunnel: w949 -> [w963 _]
      frame False {
      }
      frame True {
      }
    }
    n756 = case shown="No Error" w948 {
      selector: w948 -> [w969 w1295]
      tunnel: [w974 w1300] -> w962
      tunnel: [w973 w1292] -> w961
      tunnel: w951 -> [w972 w1298]
      tunnel: w960 -> [w971 w1297]
      tunnel: [w970 w1297] -> w959
      frame No Error {
        n757 = stacked-sequence {
          tunnel: [w984 _ _ _ _ _] -> w974
          tunnel: [w983 _ _ _ _ _] -> w973
          tunnel: w972 -> [w979 _ _ _ _ _]
          tunnel: w969 -> [w978 _ _ _ _ _]
          tunnel: w971 -> [_ w1092 _ _ _ _]
          tunnel: [_ w1091 _ _ _ _] -> w970
          tunnel: [_ w1063 _ _ _ _] -> _
          frame #0 {
            n758 = property class="Instr"(reference=w979, error in=w978) -> (reference out=w981:refnum<visa-resource-name>, error out=w982:errorcluster, "Serial Settings:Number of Bytes at Serial Port"=w975:u32)
            "Sps 3" <- w975
            "Port 1" <- w975
            n759 = Greater?(x=w975, y=u32 5) -> (0:w977:bool)
            n760 = case shown="True" w977 {
              tunnel: w981 -> [w986 w1007]
              tunnel: w982 -> [w985 w1008]
              tunnel: [w985 w1010] -> w983
              tunnel: [w986 w1009] -> w984
              frame False {
              }
              frame True {
                # "Out as Volts"
                n761 = local read "Residual Uno"() -> (w1001:string)
                n762 = while {
                  tunnel: [w1047] -> w1010
                  tunnel: [w1046] -> w1009
                  tunnel: w1008 -> [w1045]
                  tunnel: w1007 -> [w1044]
                  tunnel: [w1041] -> _
                  shift-right: [w1037] -> w989
                  shift-left: w1001 -> [w1039]
                  i -> [w1041]
                  stop <- w1042 stop-if-true
